vi "AxisReadValues_Write.vi"(1 "AxisReadValuesIN":T1, 2 "AxisNo":u16) -> ()   [LabVIEW 2020, in "SMCD14_lib.lvlib"]
uses:
  SMCD14_lib.lvlib
  AxisReadValues_typedef.ctl
  Globals.vi
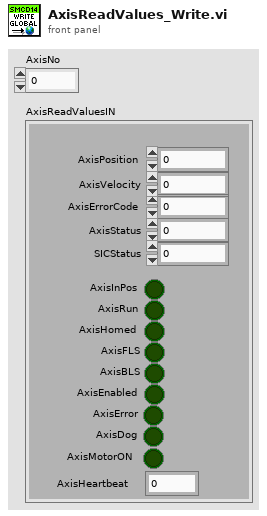
[diagram p1: front panel]
types:
  T1 = typedef "SMCD14_lib.lvlib/AxisReadValues_typedef.ctl" = cluster{"AxisPosition":dbl, "AxisStatus":i16, "AxisErrorCode":i16, "AxisInPos":bool, "AxisRun":bool, "AxisHomed":bool, "AxisFLS":bool, "AxisBLS":bool, "AxisEnabled":bool, "AxisError":bool, "AxisDog":bool, "AxisVelocity":dbl, "AxisHeartbeat":i16, "SICStatus":i16, "AxisMotorON":bool}
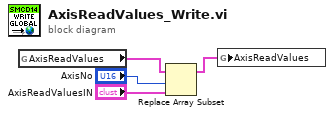
[diagram p0: block diagram]
diagram:
  n1 = global read "Globals.vi" "AxisReadValues"() -> (w4:T1[])
  n2 = Replace Array Subset(array=w4, new element="AxisReadValuesIN", index="AxisNo") -> (w3:T1[])
  n3 = global write "Globals.vi" "AxisReadValues"(w3) -> ()
